vi "PH_ImageOperator.Set Energy Unit.vi"(0 "i ref in":refnum<vi>, 5 "error in (no error)":errorcluster) -> (14 "i ref out":refnum<vi>, 19 "error out":errorcluster)   [LabVIEW 2014, in "PH_ImageOperator.lvlib"]
doc: "This VI chercks some states and sets - depending on this - the energy unit (in case of a change) to own attributes and the GUI element."
uses:
  PH_ImageOperator.lvlib
  PH_Basics/PH_StatusHandler/PH_StatusHandler.Status.ctl
  PH_Basics/PH_Img_BaseClass/PH_Img_BaseClass.lvlib
  PH_Basics/PH_StatusHandler/PH_StatusHandler.lvlib
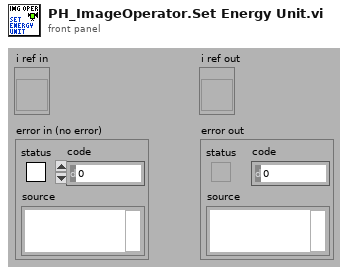
[diagram p1: front panel]
types:
  T1 = typedef "PH_StatusHandler.lvlib/PH_StatusHandler.Status.ctl" = i16
  T2 = typedef "PH_ImageOperator.lvlib/PH_ImageOperator.i attribute.ctl" = cluster{"GUI Refs":cluster{"Delete":refnum<vi>, "Calibration status":refnum<vi>, "BI subtracted":refnum<vi>, "calc Energy":refnum<vi>, "Energy: expected value":refnum<vi>, "Energy: Tolerance":refnum<vi>, "Energy calculated":refnum<vi>, "Energy":refnum<vi>, "calc Beam Anal":refnum<vi>, "Maj Diam 1/esquare":refnum<vi>, "Min Diam 1/esquare":refnum<vi>, "Azi Angle":refnum<vi>, "Min/Maj Diam esquare":refnum<vi>, "Beam analysed":refnum<vi>, "CoG - x":refnum<vi>, "CoG - y":refnum<vi>, "BA: Method":refnum<vi>, "BA: Steps":refnum<vi>, "BA: Factor":refnum<vi>, "calc Traces":refnum<vi>, "Traces: Fit Gauss":refnum<vi>, "Traces calculated":refnum<vi>, "Maj FWHM":refnum<vi>, "Min FWHM":refnum<vi>, "Major Trace":refnum<vi>, "Minor Trace":refnum<vi>, "Maj Fit Order":refnum<vi>, "Min Fit Order":refnum<vi>, "Position calculated":refnum<vi>, "Position":refnum<vi>, "Type":refnum<vi>, "Center":refnum<vi>, "exp - X":refnum<vi>, "exp - Y":refnum<vi>, "Tolerance":refnum<vi>, "f":refnum<vi>, "M":refnum<vi>, "D":refnum<vi>, "q":refnum<vi>, "Dummy Method":refnum<vi>, "Dummy Type":refnum<vi>, "Global On":refnum<vi>, "Traces: No offset":refnum<vi>, "Maj 99%":refnum<vi>, "Min 99%":refnum<vi>, "GUI FF Image":refnum<vi>, "calc Fill Factor":refnum<vi>, "FF calculated":refnum<vi>, "Fill Factor: Filter?":refnum<vi>, "FF: Damage Threshold":refnum<vi>, "FF: Threshold":refnum<vi>, "FF: max allow. Energy":refnum<vi>, "FF: Fillfactor":refnum<vi>, "Calibration data":refnum<vi>}, "List of GUIs":string[], "Calibration":cluster{"Status":T1, "Calibration data":T3, "Calibration Data File":path}, "Final Image":cluster{"BI Subtraction Failure":bool}, "Energy":cluster{"on":bool, "expected value [mJ]":dbl, "Tolerance [%]":dbl, "State":T1, "Energy [mJ]":dbl, "Unit":string, "calculated @":timestamp}, "Beam Analysis":cluster{"on":bool, "Data":T4, "Method":bool, "Steps":i32, "Factor":i32, "ROI":cluster{"Left":i32, "Top":i32, "Right":i32, "Bottom":i32}, "analysed @":timestamp}, "Trace Analysis":cluster{"on":bool, "Fit on":bool, "Maj FWHM":dbl, "Min FWHM":dbl, "Maj Fit Order":i32, "Min Fit Order":i32, "No Offset":bool, "Maj 99%":dbl, "Min 99%":dbl, "Traces":cluster{"XScaleName":string, "Y Scale Minimum":sgl, "Y Scale Maximum":sgl, "X Scale Minimum":sgl, "X Scale Maximum":sgl, "Traces":cluster{"Index":sgl[], "Trace":dbl[]}[]}[], "analysed @":timestamp}, "Position Analysis":cluster{"on":bool, "exp - X":i32, "exp - Y":i32, "focal length [mm]":dbl, "Magnification":dbl, "Delta":dbl, "Theta":dbl, "Tolerance":dbl, "Type":bool, "analysed @":timestamp}, "Fill Factor":cluster{"on":bool, "Filter on?":bool, "Threshold":dbl, "Damage Threshold [J/cm²]":dbl, "Fillfactor":dbl, "Max. allowed Energy [J]":dbl, "calculated @":timestamp}, "Statistician Service ID":i32, "Images":cluster{"Background":T5, "OP":T5, "GUI":T5, "BA: ROI":T5, "Trace: Turn":T5, "FF: Main":T5, "FF: Help":T5, "PSDB: BG":T5, "PSDB: OP":T5, "PSDB: FF":T5}}
  T3 = typedef "PH_ImageCalibrator.lvlib/PH_ImageCalibrator.Calibration Data.ctl" = cluster{"Date":string, "Time":string, "Cam Settings":cluster{"Cam ID":string, "Gain":dbl, "Brightness":dbl, "Shutter":dbl, "Cam Error":bool, "Mode":i32}, "Background Image":cluster{"Image":dbl[][], "Image Error":bool}, "Linear Calibration":cluster{"Calibration Factor":dbl, "not mm or mrad":bool}, "Energy Calibration":cluster{"Calibration Factor":dbl, "no mJ":bool}}
  T4 = typedef "PH_ImageOperator.lvlib/PH_ImageOperator.Beam Analysis Data.ctl" = cluster{"CoG-x":sgl, "CoG-y":sgl, "Maj Dim":dbl, "Min Dim":dbl, "Ellipticity":dbl, "Azimuth Angle [rad]":dbl, "Azi Angle rel to Maj?":bool}
  T5 = typedef "IMAQ Image.ctl" = refnum<image>
  T6 = typedef "PH_Img_BaseClass.lvlib/PH_Img_BaseClass.i attribute.ctl" = cluster{"GUI Refs":T7, "Timeout Image [ms]":i32, "Default Periodic Period [ms]":i32, "Camera":cluster{"Instancename":string, "Notifier":refnum<notifier>}, "Palette":T8, "Cam Settings":cluster{"Cam ID":string, "Gain":dbl, "Brightness":dbl, "Shutter":dbl, "Cam Info Failure":bool, "Mode":i32}}
  T7 = typedef "PH_Img_BaseClass.lvlib/PH_Img_BaseClass.GUI Refs.ctl" = cluster{"Timeout":refnum<vi>, "Image":refnum<vi>, "Palette":refnum<vi>, "Timeout Set":refnum<vi>}
  T8 = typedef "PH_Img_BaseClass.lvlib/PH_Img_BaseClass.Palette.ctl" = i32
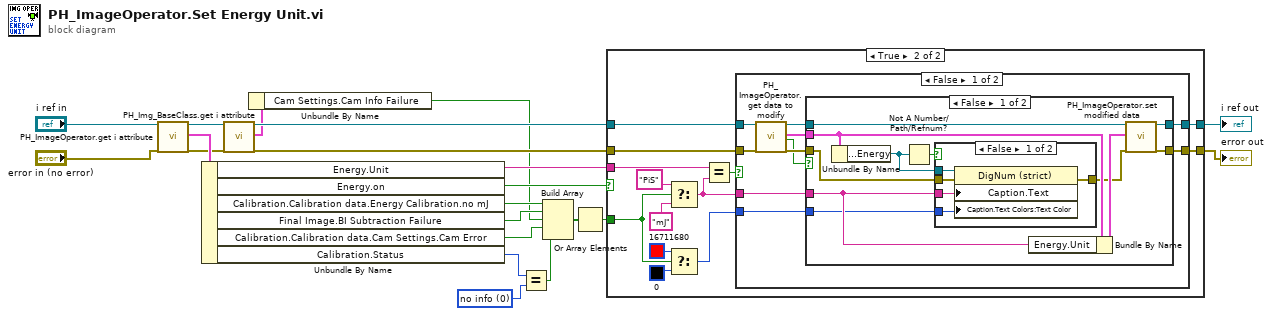
[diagram p0: block diagram]
diagram:
  w7 = T1 0 items=["no info", "off/false/out", "on/true/in", "Failure", "Alarm", "Status 1", "Status 2", "Status 3"] ("Calibration.Status")
  n1 = call "PH_ImageOperator.get i attribute.vi"("i ref in"="i ref in", "error in (no error)"="error in (no error)") -> ("i ref out"=w17:refnum<vi>, "i attribute"=w16:T2, "error out"=w4:errorcluster)  [unwired: 15 in]
  n2 = Unbundle By Name(w16) -> ("Energy.Unit"=w21:string, "Energy.on"=w20:bool, "Calibration.Calibration data.Energy Calibration.no mJ"=w13:bool, "Final Image.BI Subtraction Failure"=w12:bool, "Calibration.Calibration data.Cam Settings.Cam Error"=w9:bool, "Calibration.Status"=w8:T1)
  n3 = call "PH_Img_BaseClass.get i attribute.vi"("i ref in"=w17, "error in (no error)"=w4) -> ("i ref out"=w5:refnum<vi>, "i attribute"=w2:T6, "error out"=w3:errorcluster)  [unwired: 15 in]
  n4 = Unbundle By Name(w2) -> ("Cam Settings.Cam Info Failure"=w1:bool)
  n5 = Equal?(x=w8, y=w7) -> (x = y?=w6:bool)
  n6 = Build Array(w13, w12, w1, w9, w6) -> (w11:bool[])
  n7 = Or Array Elements(Boolean array=w11) -> (logical OR=w10:bool)
  n8 = case shown="True" w20 {
    tunnel: w5 -> [w23 w36]
    tunnel: w3 -> [w22 w35]
    tunnel: [w23 w34] -> w18
    tunnel: [w22 w33] -> w19
    tunnel: w21 -> [_ w32]
    tunnel: w10 -> [_ w26]
    frame False {
    }
    frame True {
      n9 = Select(t="PiS", s=w26, f="mJ") -> (s? t:f=w30:string)
      n10 = Select(t=u32 16711680 ("Color"), s=w26, f=u32 0 ("Color")) -> (s? t:f=w27:u32)
      n11 = Equal?(x=w32, y=w30) -> (x = y?=w31:bool)
      n12 = case shown="False" w31 {
        tunnel: w36 -> [w43 w67]
        tunnel: w35 -> [w42 w66]
        tunnel: [w41 w67] -> w34
        tunnel: [w40 w66] -> w33
        tunnel: w30 -> [w38 _]
        tunnel: w27 -> [w37 _]
        frame False {
          n13 = call "PH_ImageOperator.get data to modify.vi"("i ref in"=w43, "error in (no error)"=w42) -> ("i ref out"=w45:refnum<vi>, "i attribute"=w44:T2, "timed out"=w39:bool, "error out"=w46:errorcluster)  [unwired: 14 in]
          n14 = case shown="False" w39 {
            tunnel: w46 -> [w48 w64]
            tunnel: w45 -> [w57 w65]
            tunnel: [w56 w65] -> w41
            tunnel: [w55 w64] -> w40
            tunnel: w44 -> [w54 _]
            tunnel: w38 -> [w50 _]
            tunnel: w37 -> [w47 _]
            frame False {
              n15 = Unbundle By Name(w54) -> ("GUI Refs.Energy"=w51:refnum<vi>)
              n16 = Not A Number/Path/Refnum?(number/path/refnum=w51) -> (NaN/Path/Refnum?=w52:bool)
              n17 = case shown="False" w52 {
                tunnel: w48 -> [w62 w63]
                tunnel: [w61 w63] -> w49
                tunnel: w51 -> [w60 _]
                tunnel: w50 -> [w59 _]
                tunnel: w47 -> [w58 _]
                frame False {
                  n18 = property class="DigNum (strict)"(reference=w60, error in=w62, "Caption.Text"=w59, "Caption.Text Colors:Text Color"=w58) -> (error out=w61:errorcluster)  [unwired: 1 out]
                }
                frame True {
                }
              }
              n19 = Bundle By Name(cluster=w54, "Energy.Unit"=w50) -> (w53:T2)
              n20 = call "PH_ImageOperator.set modified data.vi"("i ref in"=w57, "i attribute"=w53, "error in (no error)"=w49) -> ("i ref out"=w56:refnum<vi>, "error out"=w55:errorcluster)  [unwired: 15 in]
            }
            frame True {
            }
          }
        }
        frame True {
        }
      }
    }
  }
  "error out" <- w19
  "i ref out" <- w18
